vi "Configure Tx Channel.vi"(8 "error in":errorcluster, 9 "labels settings for RT":T1[](array[typedef]) {"Label Timestamp Channel Data Reference" format="%.0x"; "Word Initial Raw Value" format="%032.0f"; "Label Disable/Trigger Channel Reference" format="%.0x"; "parameter driver data"."Tx parameter refs" format="%.0x"; "SDI" format="%02b"; "label" format="%.0o"}, 10 "channel number in":u8, 11 "board handle in":u8) -> (0 "error out":errorcluster, 2 "channel number out":u8, 3 "board handle out":u8)   [LabVIEW 2020, in "AIM ARINC 429 Hardware API.lvlib"]
doc: "Configures all of the labels for a specified channel to be received."
uses:
  AIM ARINC 429 Hardware API.lvlib
  Shared/RT Label Settings.ctl
  Shared/Label.ctl
  Shared/RT Parameters.ctl
  Shared/Parameter Definition.ctl
  <vilib>/NI/NI VeriStand Encoding and Decoding/Encoding.ctl
  <vilib>/NI VeriStand/Custom Device API/Custom Device Item Ref.ctl
  Shared/Transfer Type.ctl
  <vilib>/NI VeriStand/Custom Device API/Data Reference.ctl
  <instrlib>/AIM GmbH/_ARINC-429/subvi/Error Converter (ErrCode or Status).vi
  <instrlib>/AIM GmbH/_ARINC-429/subvi/Get Library Path.vi
  <instrlib>/AIM GmbH/_ARINC-429/VIs/Library/Api429Lib Error Desc Get.vi
  <instrlib>/AIM GmbH/_ARINC-429/subvi/Get Error Number Offset.vi
  <vilib>/Utility/error.llb/Error Cluster From Error Code.vi
  <instrlib>/AIM GmbH/_ARINC-429/AIM429LV.lvlib
  <vilib>/NI/NI VeriStand Encoding and Decoding/Encoding and Decoding.lvlib
  <vilib>/NI VeriStand/Custom Device API/Custom Device API.lvlib
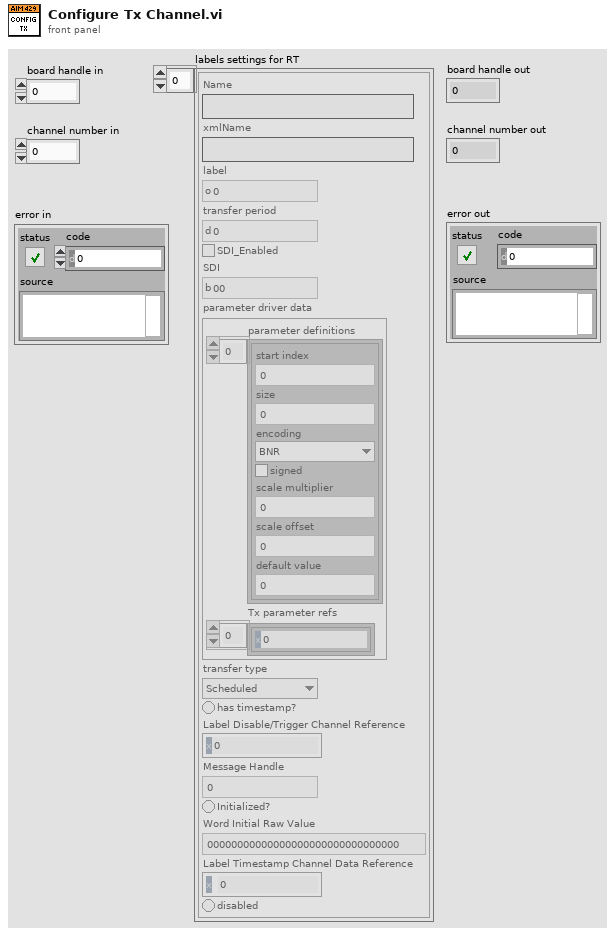
[diagram p1: front panel]
types:
  T1 = typedef "RT Label Settings.ctl" = cluster{"Name":string, "xmlName":string, "label":T2, "transfer period":u32, "SDI_Enabled":bool, "SDI":u8, "parameter driver data":T3, "transfer type":T7, "has timestamp?":bool, "Label Disable/Trigger Channel Reference":T6, "Message Handle":u64, "Initialized?":bool, "Word Initial Raw Value":u32, "Label Timestamp Channel Data Reference":T8, "disabled":bool}
  T2 = typedef "Label.ctl" = u8
  T3 = typedef "RT Parameters.ctl" = cluster{"parameter definitions":T4[], "Tx parameter refs":T6[]}
  T4 = typedef "Parameter Definition.ctl" = cluster{"start index":i32, "size":i32, "encoding":T5, "signed":bool, "scale multiplier":dbl, "scale offset":dbl, "default value":dbl}
  T5 = typedef "Encoding and Decoding.lvlib/Encoding.ctl" = enum16{"BNR", "BCD", "Discrete"}
  T6 = typedef "Custom Device API.lvlib/Custom Device Item Ref.ctl" = u64
  T7 = typedef "Transfer Type.ctl" = enum16{"Scheduled", "Acyclic", "Block", "Strobe"}
  T8 = typedef "Custom Device API.lvlib/Data Reference.ctl" = i32
  T9 = cluster{"xfer_id":u32, "xfer_type":u32, "err_type":u32, "xfer_gap":u16, "ir_index":u16, "buf_size":u16, "xfer_ir":u8}
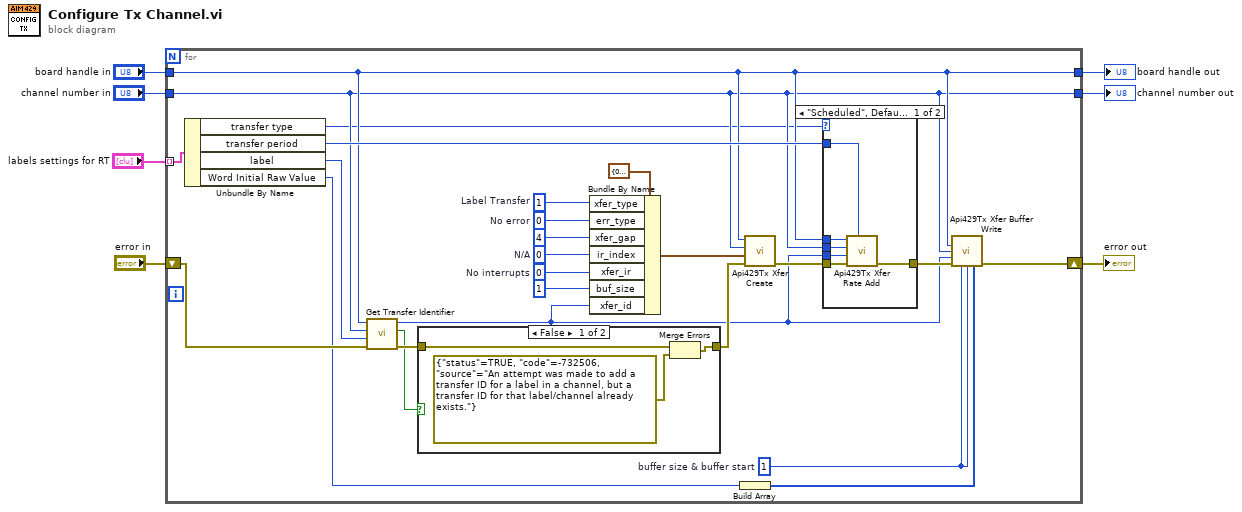
[diagram p0: block diagram]
diagram:
  n1 = for {
    tunnel: "channel number in" -> [w21]
    shift-right: [w14] -> w5
    shift-left: "error in" -> [w32]
    tunnel: "labels settings for RT" -> [w25] mode=indexing
    tunnel: [w21] -> w3
    tunnel: "board handle in" -> [w22]
    tunnel: [w22] -> w1
    w11 = u16 1  # buffer size & buffer start
    w26 = u8 0  # No interrupts
    w28 = u16 0  # N/A
    w30 = u32 0  # No error
    w31 = u32 1  # Label Transfer
    n2 = Unbundle By Name(w25) -> ("transfer type"=w8:T7, "transfer period"=w24:u32, "label"=w18:T2, "Word Initial Raw Value"=w19:u32)
    n3 = call "Get Transfer Identifier.vi"("error in"=w32, "label number in"=w18, "channel number in"=w21, "board number in"=w22) -> ("error out"=w20:errorcluster, "new entry created"=w12:bool, "Transfer ID out"=w13:u32)  [unwired: 5 in]
    n4 = case shown="False" w12 {
      tunnel: w20 -> [w42 w43]
      tunnel: [w41 w43] -> w17
      frame False {
        n5 = Merge Errors(w42, errorcluster {"status"=TRUE, "code"=-732506, "source"="An attempt was made to add a transfer ID for a label in a channel, but a transfer ID for that label/channel already exists."} ("error constant")) -> (w41:errorcluster)
      }
      frame True {
      }
    }
    n6 = Bundle By Name(cluster=T9 {"xfer_id"=0, "xfer_type"=1, "err_type"=0, "xfer_gap"=0, "ir_index"=0, "buf_size"=0, "xfer_ir"=0} ("px_Xfer"), "xfer_type"=w31, "err_type"=w30, "xfer_gap"=u16 4 ("transfer gap in bits"), "ir_index"=w28, "xfer_ir"=w26, "buf_size"=u16 1 ("buffer size"), "xfer_id"=w13) -> (w10:T9)
    n7 = Build Array(w19) -> (w23:u32[])
    n8 = call <instrlib>:"Api429Tx Xfer Create.vi"("error in (no error)"=w17, "px_Xfer"=w10, "b_Chn"=w21, "board_handle"=w22) -> ("error out"=w16:errorcluster)  [unwired: 6 in, 1 out]
    n9 = case shown="\"Scheduled\", Default" w8 {
      tunnel: w24 -> [w38 _]
      tunnel: w22 -> [w37 _]
      tunnel: w21 -> [w36 _]
      tunnel: w16 -> [w35 w39]
      tunnel: [w34 w39] -> w15
      tunnel: w13 -> [w33 _]
      frame "Scheduled", Default {
        n10 = call <instrlib>:"Api429Tx Xfer Rate Add.vi"("ulRateInMs"=w38, "error in (no error)"=w35, "ulXferId"=w33, "ucChannel"=w36, "board_handle"=w37) -> ("error out"=w34:errorcluster)  [unwired: 6 in]
      }
      frame "Acyclic" {
      }
    }
    n11 = call <instrlib>:"Api429Tx Xfer Buffer Write.vi"("board_handle"=w22, "b_Chn"=w21, "ul_XferId"=w13, "error in (no error)"=w15, "w_BufStart"=w11, "w_BufSize"=w11, "pl_LData"=w23) -> ("error out"=w14:errorcluster)  [unwired: 8 in]
  }
  "board handle out" <- w1
  "channel number out" <- w3
  "error out" <- w5
